vi "get statistics_dataview.vi"(8 "Y-column names":string[](array[string])=["mr"], 10 "column extension":string[](array[string])=["022", "016"], 11 "Graph array":cluster{"output":dbl[], "output":dbl[]}[](array[cluster])=[{"output"=array[5704 elements], "output"=array[5704 elements]}, {"output"=array[27359 elements], "output"=array[27359 elements]}]) -> ()   [LabVIEW 2020]
uses:
  <vilib>/gmath/NI_Gmath.lvlib
panel:
  out "String":string
  in  "file path (dialog if empty)":path
  in  "plot":enum16{"mean", "spreadness"}(ring)
  out "XY Graph":cluster{dbl[], dbl[]}(graph)
  in  "std type":i32(ring) items=["standard deviation", "range", "mean absolute deviation", "interquartile range"]
  in  "mean type":T1(ring)
  in  "export":T2(ring)=enum."write to clipboard"
  in  "stop":bool=TRUE
  in  "export data":bool
  # "Report mean and std values for the graph arrays"
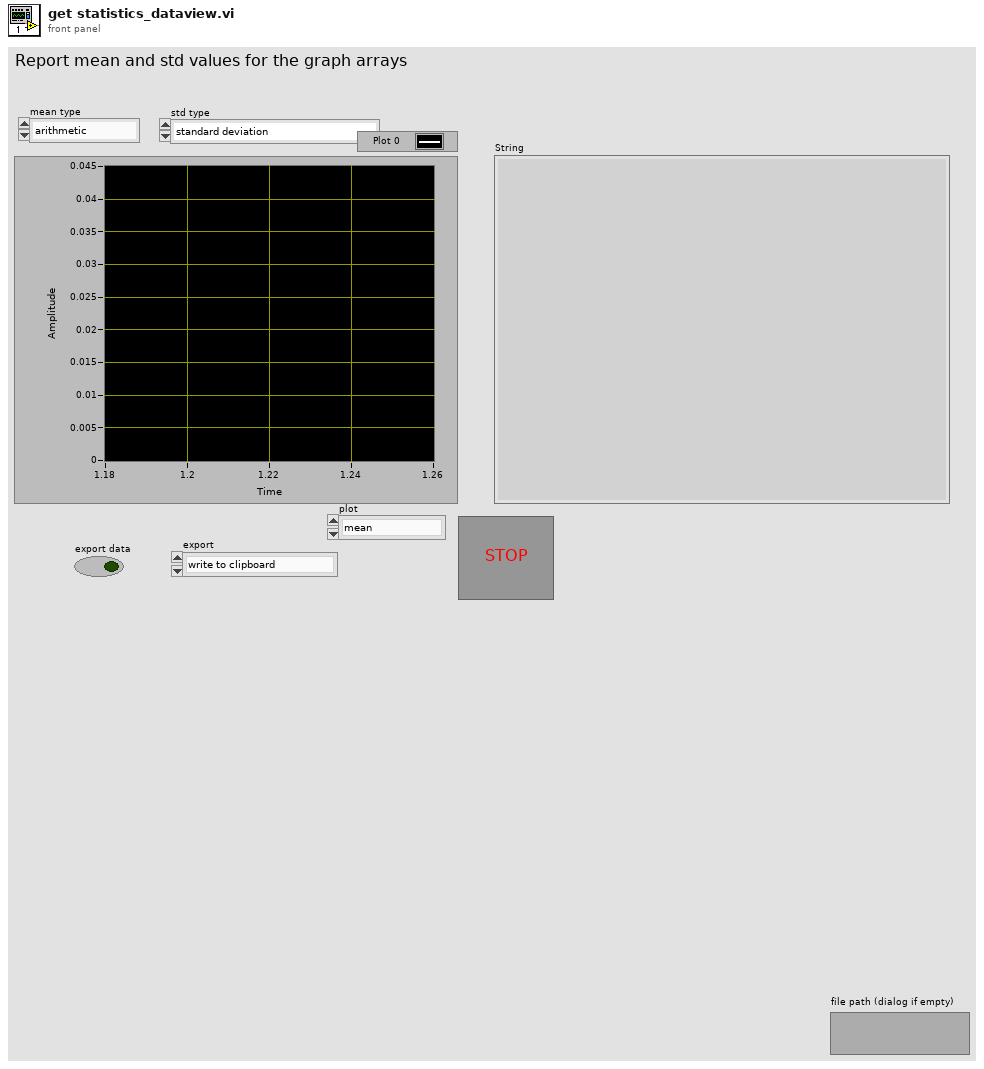
[diagram p1: front panel]
types:
  T1 = enum16{"arithmetic", "geometric", "harmonic", "trimmed", "median"}
  T2 = enum16{"Save as Ascill file", "write to clipboard"}
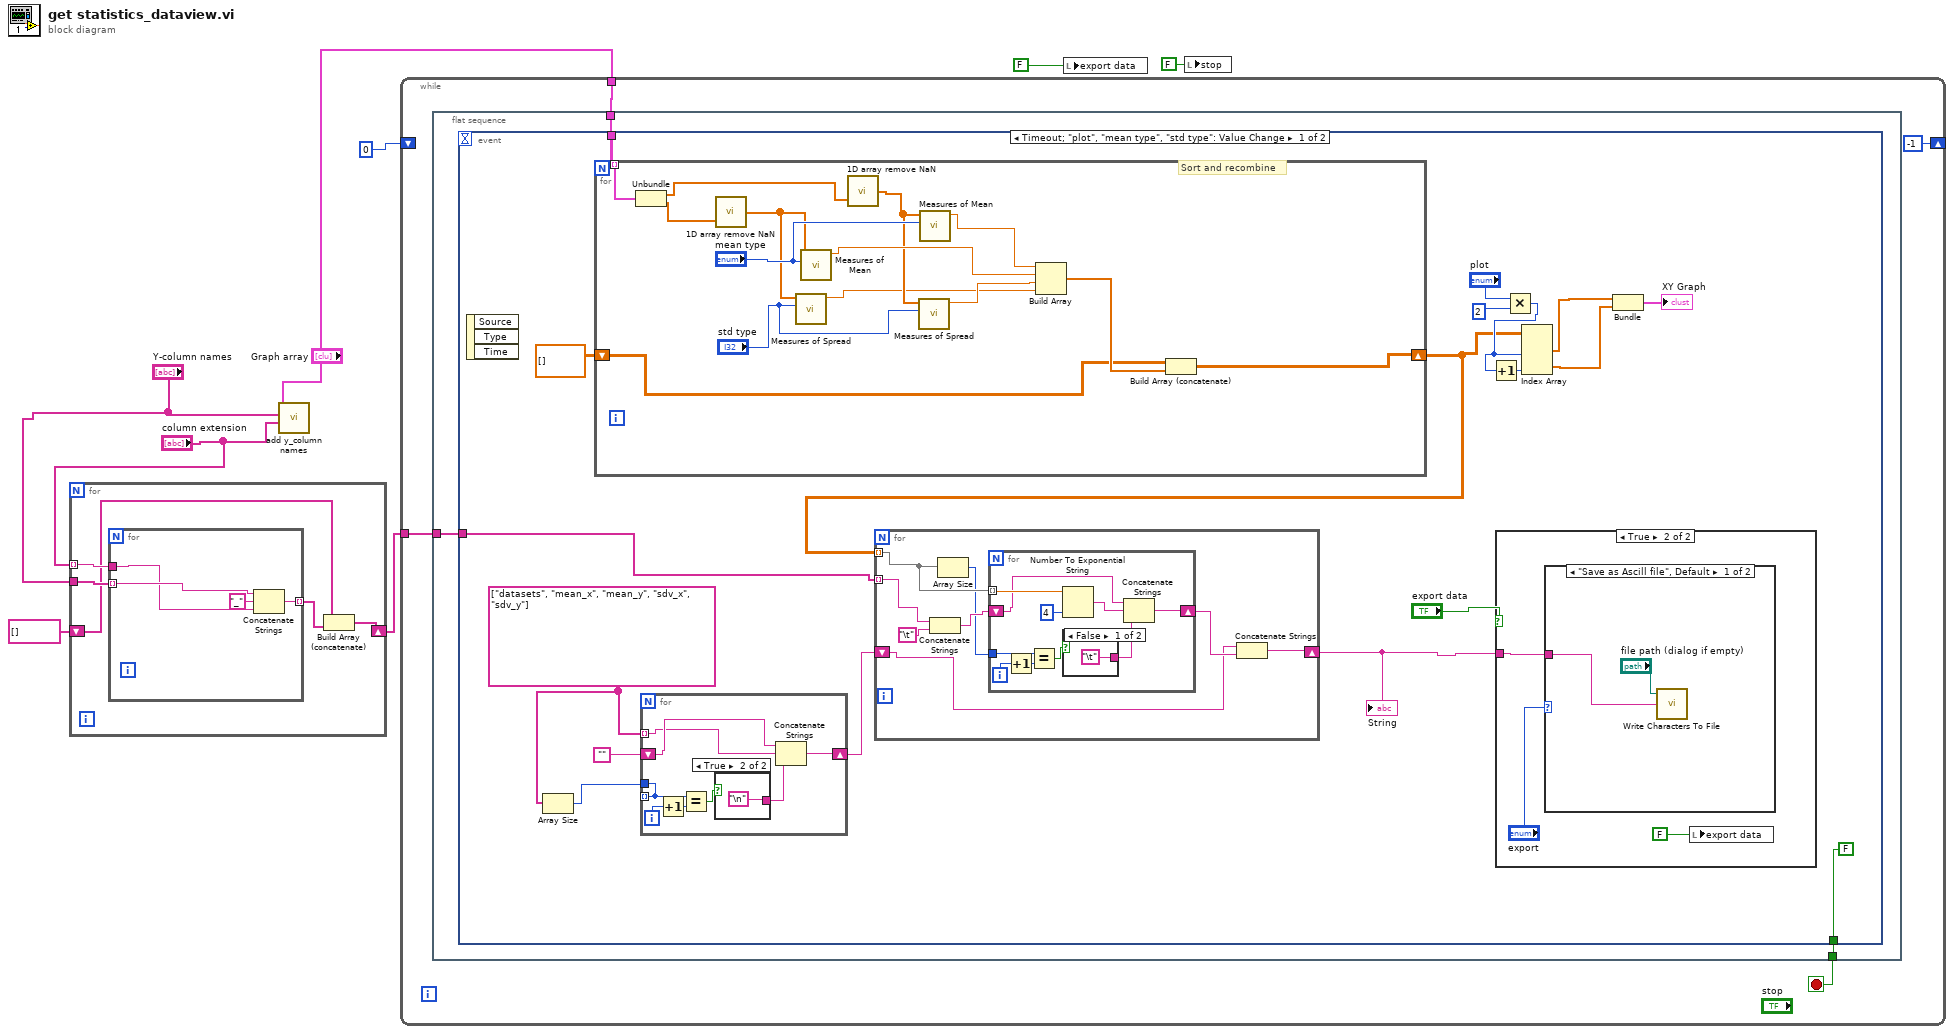
[diagram p0: block diagram]
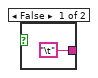
[diagram p2: hidden frame]
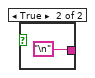
[diagram p3: hidden frame]
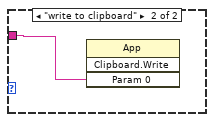
[diagram p5: hidden frame]
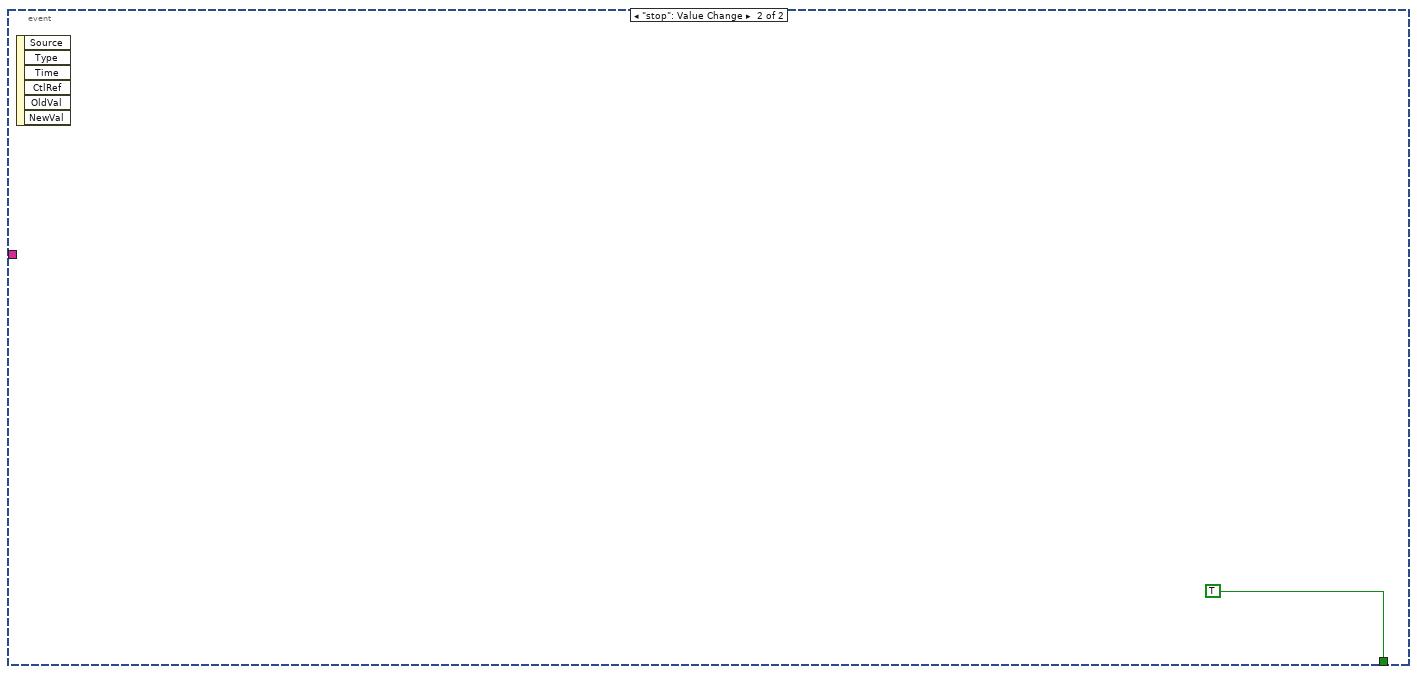
[diagram p6: hidden frame]
diagram:
  n1 = for {
    tunnel: "column extension" -> [w12] mode=indexing
    tunnel: "Y-column names" -> [w13]
    shift-right: [w9] -> w2
    shift-left: string[] [] -> [w10]
    n2 = for {
      tunnel: w13 -> [w17] mode=indexing
      tunnel: w12 -> [w15]
      tunnel: [w14] -> w11 mode=indexing
      n3 = Concatenate Strings(w17, "_" ("string"), w15) -> (w14:string)
    }
    n4 = Build Array (concatenate)(w10, w11) -> (w9:string[])
  }
  n5 = call "add y_column names.vi"("column extension"="column extension", "old y-column names"="Y-column names", "graph file"="Graph array") -> ()  [unwired: 6 in, 3 out]
  n6 = while {
    tunnel: "Graph array" -> [w21]
    tunnel: w2 -> [w19]
    shift-right: [-1] -> _
    shift-left: 0 -> [_]
    stop <- w20 stop-if-true
    n7 = flat-sequence {
      tunnel: w21 -> [w24]
      tunnel: [w23] -> w20
      tunnel: w19 -> [w22]
      frame #0 {
        n8 = event shown="[0] Timeout;  \"plot\", \"mean type\", \"std type\": Value Change" {
          selector: _ -> [_ _]
          dyn-events: _ -> [_ _]
          timeout: _ -> [_ _]
          tunnel: w24 -> [w41 _]
          tunnel: [FALSE ("stop (press twice)") TRUE ("stop (press twice)")] -> w23
          tunnel: w22 -> [w29 _]
          event Timeout; "plot", "mean type", "std type": Value Change {
            w28 = string[] ["datasets", "mean_x", "mean_y", "sdv_x", "sdv_y"] ("Y-column names")
            n9 = event-data() -> ()  [unwired: 1 in, 3 out]
            n10 = Array Size(array=w28) -> (size(s)=w27:i32)
            n11 = for {
              tunnel: w41 -> [w86] mode=indexing
              shift-right: [w75] -> w31
              shift-left: dbl[][] [] -> [w74]
              # "Sort and recombine"
              n12 = Unbundle(w86) -> ("output"=w84:dbl[], "output"=w85:dbl[])
              n13 = call "1D array remove NaN.vi"("Array input"=w85) -> ("cleaned array"=w73:dbl[])  [unwired: 1 in]
              n14 = call <vilib>:"Measures of Spread.vi"("type"="std type", "x array"=w73) -> ("spread value"=w77:dbl)  [unwired: 8 in, 1 out]
              n15 = call <vilib>:"Measures of Mean.vi"("type"="mean type", "x array"=w73) -> ("mean value"=w80:dbl)  [unwired: 8 in, 1 out]
              n16 = call "1D array remove NaN.vi"("Array input"=w84) -> ("cleaned array"=w79:dbl[])  [unwired: 1 in]
              n17 = call <vilib>:"Measures of Spread.vi"("type"="std type", "x array"=w79) -> ("spread value"=w78:dbl)  [unwired: 8 in, 1 out]
              n18 = call <vilib>:"Measures of Mean.vi"("type"="mean type", "x array"=w79) -> ("mean value"=w81:dbl)  [unwired: 8 in, 1 out]
              n19 = Build Array(w81, w80, w78, w77) -> (w76:dbl[])
              n20 = Build Array (concatenate)(w74, w76) -> (w75:dbl[][])
            }
            n21 = for {
              tunnel: w28 -> [w44] mode=indexing
              shift-right: [w49] -> w26
              shift-left: "" -> [w50]
              tunnel: [w43] -> _ mode=indexing
              tunnel: w27 -> [w43]
              i -> [w46]
              n22 = Increment(x=w46) -> (x+1=w45:i32)
              n23 = Equal?(x=w43, y=w45) -> (x = y?=w47:bool)
              n24 = case shown="True" w47 {
                tunnel: ["\t" "\n"] -> w48
                frame False {
                }
                frame True {
                }
              }
              n25 = Concatenate Strings(w50, w44, w48) -> (w49:string)
            }
            n26 = for {
              tunnel: w31 -> [w57] mode=indexing
              shift-right: [w54] -> w30
              shift-left: w26 -> [w53]
              tunnel: w29 -> [w60] mode=indexing
              n27 = Concatenate Strings(w60, "\t") -> (w59:string)
              n28 = Array Size(array=w57) -> (size(s)=w56:i32)
              n29 = for {
                tunnel: w57 -> [w70] mode=indexing
                shift-right: [w67] -> w55
                shift-left: w59 -> [w68]
                tunnel: w56 -> [w63]
                i -> [w64]
                n30 = Increment(x=w64) -> (x+1=w62:i32)
                n31 = Equal?(x=w63, y=w62) -> (x = y?=w65:bool)
                n32 = Number To Exponential String(number=w70, precision (6)=i16 4) -> (E-format string=w69:string)  [unwired: 2 in]
                n33 = case shown="False" w65 {
                  tunnel: ["\t" "\n"] -> w66
                  frame False {
                  }
                  frame True {
                  }
                }
                n34 = Concatenate Strings(w68, w69, w66) -> (w67:string)
              }
              n35 = Concatenate Strings(w53, w55) -> (w54:string)
            }
            "String" <- w30
            n36 = case shown="True" "export data" {
              tunnel: w30 -> [_ w88]
              frame False {
              }
              frame True {
                n37 = case shown="\"Save as Ascill file\", Default" "export" {
                  tunnel: w88 -> [w90 w92]
                  frame "Save as Ascill file", Default {
                    n38 = call <vilib>:"Write Characters To File.vi"("character string"=w90, "file path (dialog if empty)"="file path (dialog if empty)") -> ()  [unwired: 1 in, 3 out]
                  }
                  frame "write to clipboard" {
                    n39 = invoke class="App" method="Clipboard.Write"("Param 0"=w92) -> ()  [unwired: 3 in, 4 out]
                  }
                }
                n40 = local write "export data"(FALSE ("export spectrum")) -> ()
              }
            }
            n41 = Multiply(x="plot", y=2) -> (x*y=w35:i32)
            n42 = Increment(x=w35) -> (x+1=w38:i32)
            n43 = Index Array(array=w31, index (col) #1=w35, index (col) #2=w38) -> (element #1=w34:dbl[], element #2=w33:dbl[])  [unwired: 2 in]
            n44 = Bundle(w34, w33) -> (→"XY Graph":cluster{dbl[], dbl[]})  [unwired: 1 in]
          }
          event "stop": Value Change {
            n45 = event-data() -> ()  [unwired: 1 in, 6 out]
          }
        }
      }
    }
  }
  n46 = local write "export data"(FALSE ("export spectrum")) -> ()
  n47 = local write "stop"(FALSE ("stop")) -> ()
